vi "Plot Editor_Data to Controls & Plot.vi"(0 "Plot Editor Internal Data":T2, 1 "XYGraph in":refnum<vi>, 2 "VI Title Suffix":string, 3 "Refnum based call":bool, 5 "X Array":dbl[](array[numeric]), 7 "Y Array":dbl[](array[numeric]), 11 "error in (no error)":errorcluster, 12 "Control Refnums":refnum<vi>[](array[refnum]), 13 "Plot Style":T1, 14 "Data only (T)":bool=TRUE) -> (4 "Plot Editor Internal Data":T2, 15 "error out":errorcluster)   [LabVIEW 2019, in "Plot Editor.lvlib"]
uses:
  Plot Editor.lvlib
  Plot Editor Internal Variables.ctl
  XY Graph Plot Properties.ctl
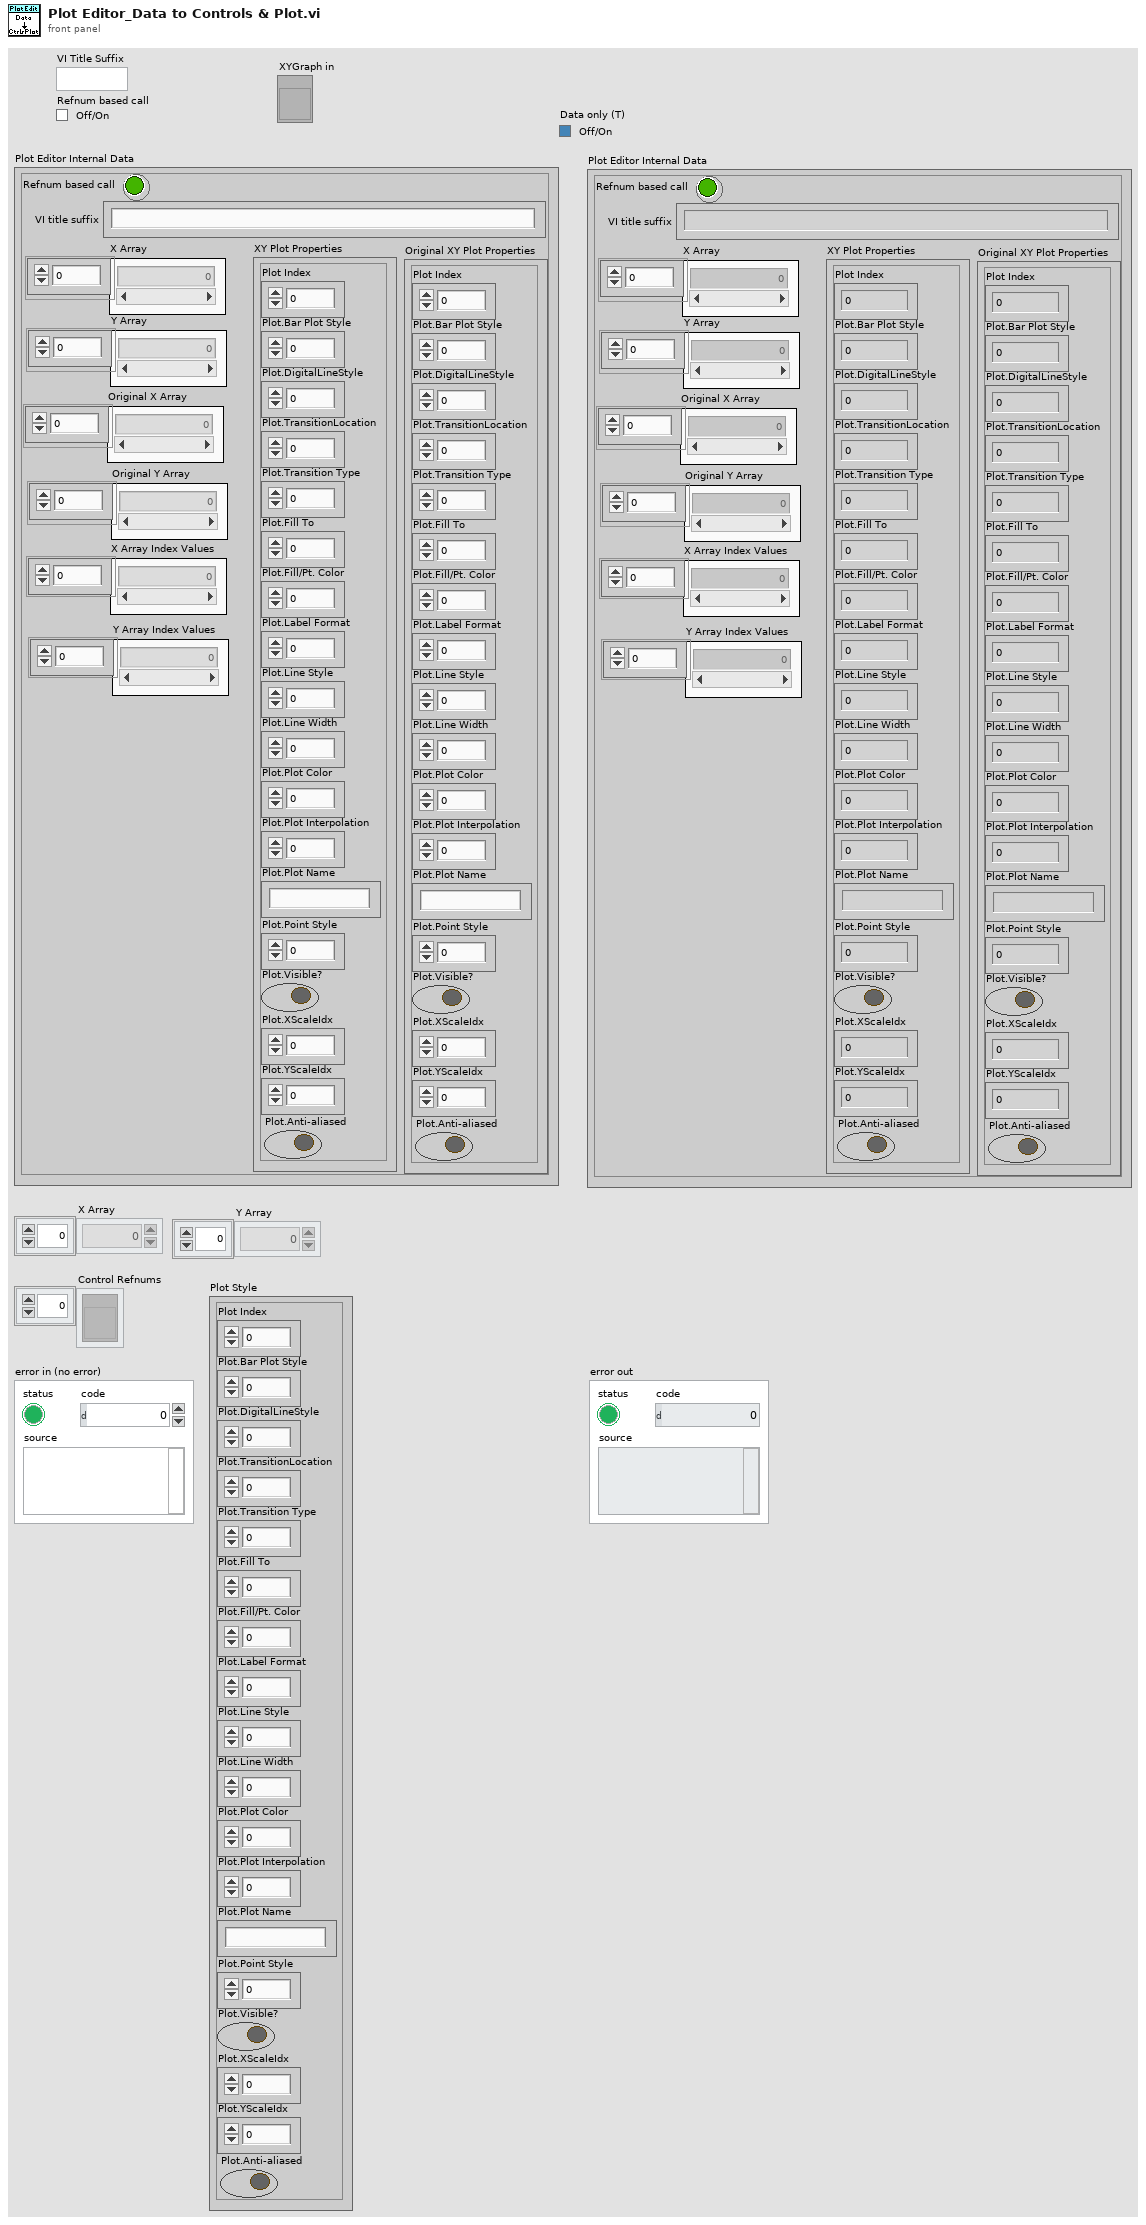
[diagram p1: front panel]
types:
  T1 = typedef "XY Graph Plot Properties.ctl" = cluster{"Plot Index":i32, "Plot.Bar Plot Style":u8, "Plot.DigitalLineStyle":u8, "Plot.TransitionLocation":u8, "Plot.Transition Type":u8, "Plot.Fill To":i16, "Plot.Fill/Pt. Color":u32, "Plot.Label Format":u8, "Plot.Line Style":u8, "Plot.Line Width":u8, "Plot.Plot Color":u32, "Plot.Plot Interpolation":u8, "Plot.Plot Name":string, "Plot.Point Style":u8, "Plot.Visible?":bool, "Plot.XScaleIdx":u32, "Plot.YScaleIdx":u32, "Plot.Anti-aliased":bool}
  T2 = typedef "Plot Editor.lvlib/Plot Editor Internal Variables.ctl" = cluster{"X Array":dbl[], "Y Array":dbl[], "XY Plot Properties":T1, "X Array Index Values":u32[], "Y Array Index Values":u32[], "Original XY Plot Properties":T1, "Original X Array":dbl[], "Original Y Array":dbl[], "VI title suffix":string, "Refnum based call":bool}
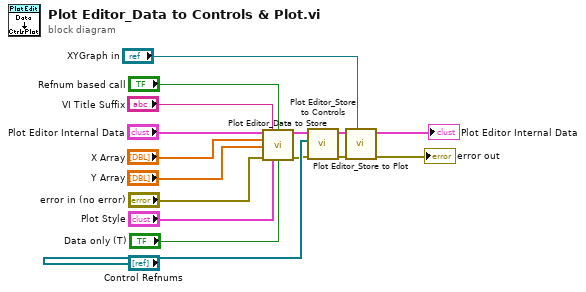
[diagram p0: block diagram]
diagram:
  n1 = call "Plot Editor_Data to Store.vi"("Plot Editor Internal Data in"="Plot Editor Internal Data", "VI Title Suffix"="VI Title Suffix", "Refnum based call"="Refnum based call", "X Array"="X Array", "Y Array"="Y Array", "Error In"="error in (no error)", "Plot Style"="Plot Style", "Data only (T: Default)/Init (F)"="Data only (T)") -> ("Plot Editor Internal Data out"=w6:T2, "Error Out"=w12:errorcluster)  [unwired: 6 in]
  n2 = call "Plot Editor_Store to Controls.vi"("Error In"=w12, "Control Refnums"="Control Refnums", "Plot Editor Internal Data in"=w6) -> ("Error Out"=w13:errorcluster, "Plot Editor Internal Data out"=w7:T2)  [unwired: 7 in]
  n3 = call "Plot Editor_Store to Plot.vi"("XYGraph in"="XYGraph in", "Error In"=w13, "Plot Editor Internal Data"=w7) -> ("Error Out"=→"error out":errorcluster, "Plot Editor Internal Data (dup)"=→"Plot Editor Internal Data":T2)  [unwired: 7 in]
